vi "Check PCC for Unintentional Islanding.vi"(8 "error in":errorcluster, 11 "On-Grid in":refnum<class "On-Grid.lvclass">) -> (0 "error out":errorcluster, 3 "On-Grid out":refnum<class "On-Grid.lvclass">)   [LabVIEW 2018, in "On-Grid Actor.lvlib" / "On-Grid.lvclass"]
uses:
  On-Grid.lvclass
  C:/Users/Administrator/Desktop/2018LabVIEW EMS/EMS Generic Actor/EMS Generic/EMS Generic.lvclass
  C:/Users/Administrator/Desktop/2018LabVIEW EMS/Optimization/Generic Optimization Actor/Generic Optimization/Generic Optimization.lvclass
  <vilib>/ORNL/CSEISMIC DDS/CSEISMIC DDS Base/Data Types/Controls/DeviceID.ctl
  <vilib>/ORNL/CSEISMIC DDS/CSEISMIC DDS Base/CSEISMIC DDS.lvclass
  Generic Optimization Actor/Generic Optimization/Generic Optimization.lvclass
  EMS Generic Actor/EMS Generic/EMS Generic.lvclass
  <vilib>/ORNL/CSEISMIC DDS/CSEISMIC DDS Base/Data Types/Controls/Generation Mode.ctl
  <vilib>/ORNL/CSEISMIC DDS/CSEISMIC DDS Base/Data Types/DER_setGenerationMode.ctl
  Device Communication and Control Abstract Actor/Device Communication and Control Abstract/Device Communication and Control Abstract.lvclass
  Utilities/Status Messaging.llb/Status Messaging.lvlib
  C:/Users/Administrator/Desktop/2018LabVIEW EMS/Device Communication and Control Abstract Actor/Device Communication and Control Abstract/Device Communication and Control Abstract.lvclass
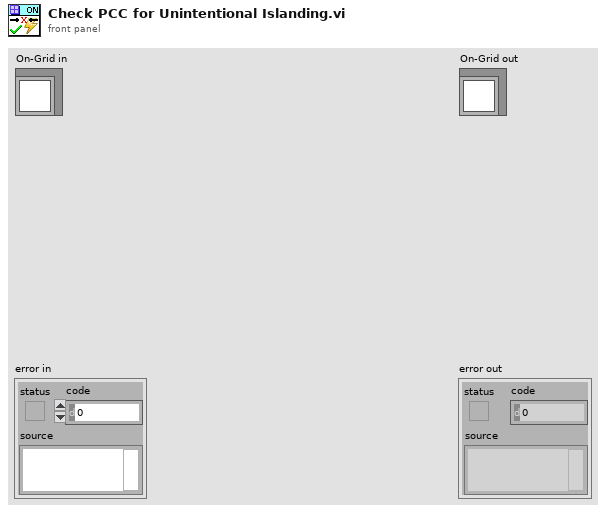
[diagram p1: front panel]
types:
  T1 = typedef "CSEISMIC DDS.lvlib/CSEISMIC DDS.lvclass/DER_setGenerationMode.ctl" = cluster{"DeviceID":T2, "Mode":T3}
  T2 = typedef "CSEISMIC DDS.lvlib/CSEISMIC DDS.lvclass/DeviceID.ctl" = string
  T3 = typedef "CSEISMIC DDS.lvlib/CSEISMIC DDS.lvclass/Generation Mode.ctl" = enum32{"Invalid", "PQ", "Droop", "PV", "PF", "VF"}
  T4 = typedef "CSEISMIC DDS.lvlib/CSEISMIC DDS.lvclass/IED_Status.ctl" = cluster{"DeviceID":T2, "Timestamp":T5, "MicrogridID":u8, "Active":bool, "Inactive":bool, "Error":i32, "Fault":bool, "ErrorString":string}
  T5 = typedef "CSEISMIC DDS.lvlib/CSEISMIC DDS.lvclass/Timestamp.ctl" = cluster{"Seconds":u64, "Remainder":u64}
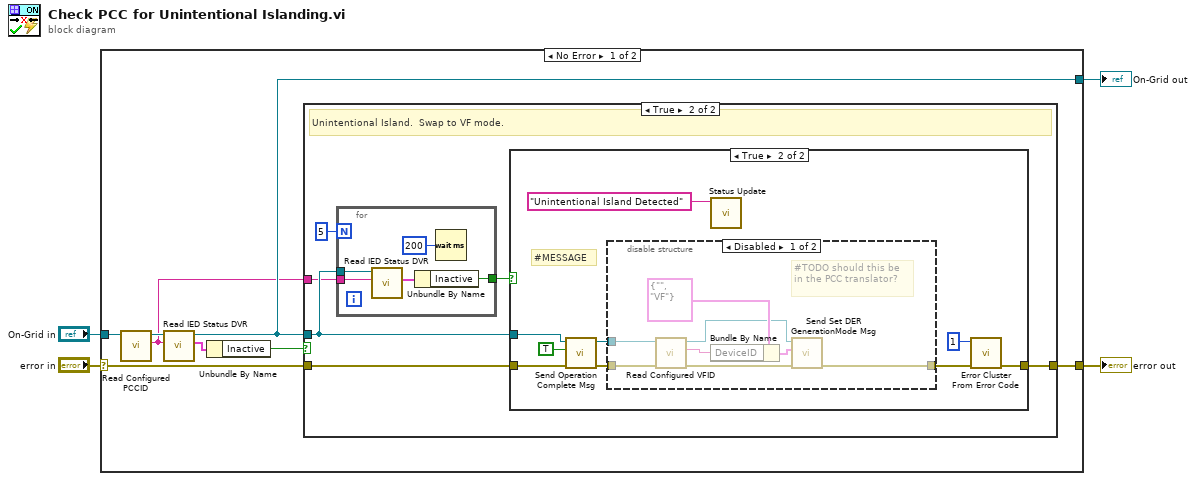
[diagram p0: block diagram]
diagram:
  n1 = case shown="No Error" "error in" {
    selector: "error in" -> [w12 w45]
    tunnel: [w11 w45] -> w3
    tunnel: [w8 w44] -> w1
    tunnel: "On-Grid in" -> [w9 w44]
    frame No Error {
      n2 = call "Read Configured PCCID.vi"("EMS Generic in"=w9) -> ("PCCID"=w5:T2, "EMS Generic out"=w6:refnum<class "On-Grid.lvclass">)  [unwired: 8 in, 1 out]
      n3 = call "Read IED Status DVR.vi"("DeviceID"=w5, "EMS Generic in"=w6) -> ("IED_Status"=w7:T4, "EMS Generic out"=w8:refnum<class "On-Grid.lvclass">)  [unwired: 6 in, 2 out]
      n4 = Unbundle By Name(w7) -> ("Inactive"=w10:bool)
      n5 = case shown="True" w10 {
        tunnel: w12 -> [w13 w18]
        tunnel: [w13 w19] -> w11
        tunnel: w8 -> [_ w17]
        tunnel: w5 -> [_ w16]
        frame False {
          # "Still on grid.  Do nothing special."
        }
        frame True {
          # "Unintentional Island.  Swap to VF mode."
          n6 = for {
            N: 5 -> [_]
            tunnel: w17 -> [w42]
            tunnel: [w41] -> w15
            tunnel: w16 -> [w40]
            n7 = call "Read IED Status DVR.vi"("DeviceID"=w40, "EMS Generic in"=w42) -> ("IED_Status"=w43:T4)  [unwired: 6 in, 3 out]
            n8 = Unbundle By Name(w43) -> ("Inactive"=w41:bool)
            n9 = Wait (ms)(milliseconds to wait=u32 200) -> ()  [unwired: 1 out]
          }
          n10 = case shown="True" w15 {
            tunnel: [w20 w29] -> w19
            tunnel: w18 -> [w20 w27]
            tunnel: w17 -> [_ w21]
            frame False {
            }
            frame True {
              # "#MESSAGE"
              n11 = call "Send Operation Complete Msg.vi"("error in"=w27, "Operation Complete"=TRUE, "Generic Optimization in"=w21) -> ("error out"=w25:errorcluster, "Generic Optimization out"=w23:refnum<class "On-Grid.lvclass">)  [unwired: 7 in]
              n12 = disable-structure shown="Disabled" {
                disable-tunnel: w25 -> [w32 w38]
                disable-tunnel: [w31 w38] -> w24
                disable-tunnel: w23 -> [w30 _]
                frame Disabled {
                  # "#TODO should this be in the PCC translator?"
                  n13 = call "Read Configured VFID.vi"("error in"=w32, "EMS Generic in"=w30) -> ("error out"=w33:errorcluster, "VFID"=w36:T2, "EMS Generic out"=w34:refnum<class "On-Grid.lvclass">)  [unwired: 7 in]
                  n14 = Bundle By Name(cluster=T1 {"DeviceID"="", "Mode"=enum."VF"} ("DER_setGenerationMode"), "DeviceID"=w36) -> (w35:T1)
                  n15 = call "Send Set DER GenerationMode Msg.vi"("error in"=w33, "DER_setGenerationMode"=w35, "SCADA Sub Abstract in"=w34) -> ("error out"=w31:errorcluster)  [unwired: 7 in, 1 out]
                }
                frame Enabled {
                }
              }
              n16 = call "Status Update.vi"("Status Update"="Unintentional Island Detected") -> ()  [unwired: 9 in, 2 out]
              n17 = call <vilib>:"Error Cluster From Error Code.vi"("error in (no error)"=w24, "error code (0)"=1) -> ("error out"=w29:errorcluster)  [unwired: 7 in]
            }
          }
        }
      }
    }
    frame Error {
    }
  }
  "error out" <- w3
  "On-Grid out" <- w1
